vi "Restart Discovery Service.vi"(8 "error in":errorcluster) -> (0 "error out":errorcluster)   [LabVIEW 2020, in "MeasurementServerTests.lvlib"]
uses:
  MeasurementServerTests.lvlib
  Runtime/MeasurementLink Measurement Server/MeasurementLink Measurement Server.lvlib
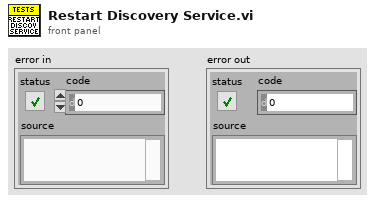
[diagram p1: front panel]
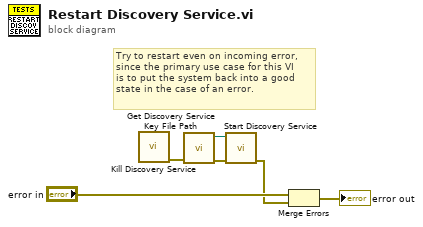
[diagram p0: block diagram]
diagram:
  # "Try to restart even on incoming error,\nsince the primary use case for this VI\nis to put the system back into a good \nstate in the case of an error."
  n1 = call "Kill Discovery Service.vi"() -> ("error out"=w5:errorcluster)  [unwired: 11 in]
  n2 = call "Get Discovery Service Key File Path.vi"("error in (no error)"=w5) -> ("error out"=w6:errorcluster, "key file path"=w1:path)  [unwired: 9 in]
  n3 = call "Start Discovery Service.vi"("error in"=w6, "key file path"=w1) -> ("error out"=w3:errorcluster)  [unwired: 9 in]
  n4 = Merge Errors("error in", w3) -> (→"error out":errorcluster)
